vi "Simulator Main.vi"() -> ()   [LabVIEW 2023]
panel:
  in  "Burn Rate (mB/t)":dbl
  in  "stop":bool
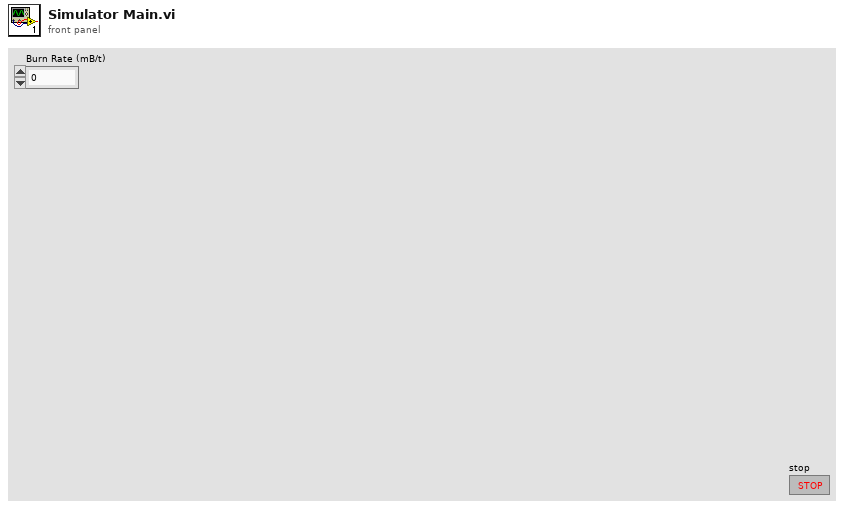
[diagram p1: front panel]
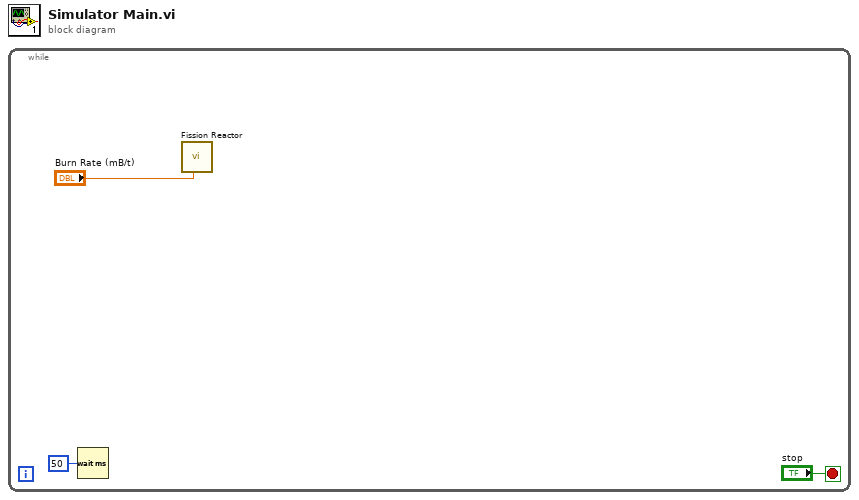
[diagram p0: block diagram]
diagram:
  n1 = while {
    stop <- "stop" stop-if-true
    n2 = Wait (ms)(milliseconds to wait=u32 50) -> ()  [unwired: 1 out]
    n3 = call "Fission Reactor.vi"("Burn Rate (mB/t)"="Burn Rate (mB/t)") -> ()  [unwired: 8 in, 3 out]
  }
